vi "Update-PV.vi"(8 "error in (no error)":errorcluster, 10 "PV":refnum<class "PV.lvclass">, 11 "CS++DIM-Client in":refnum<class "CS++DIM-Client.lvclass">) -> (0 "error out":errorcluster, 3 "CS++DIM-Client out":refnum<class "CS++DIM-Client.lvclass">)   [LabVIEW 2014, in "CS++DIM-Client.lvlib" / "CS++DIM-Client.lvclass"]
doc: "Send PV to Actor Core.vi."
uses:
  CS++DIM-Client.lvclass
  CSPP_Core/Classes/CS++ProcessVariables/ProcessVariable/PV.lvclass
  CS++DIM-Client.lvclass/CS++DIM-Client.ctl
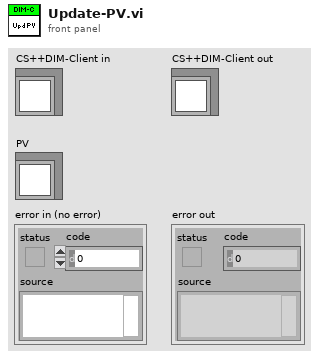
[diagram p1: front panel]
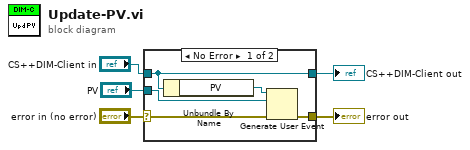
[diagram p0: block diagram]
diagram:
  n1 = case shown="No Error" "error in (no error)" {
    selector: "error in (no error)" -> [w7 w12]
    tunnel: [w6 w12] -> w4
    tunnel: [w10 w11] -> w2
    tunnel: "CS++DIM-Client in" -> [w10 w11]
    tunnel: "PV" -> [w8 _]
    frame No Error {
      n2 = Unbundle By Name(w10) -> ("PV"=w9:refnum<user-event>)
      n3 = Generate User Event(user event=w9, event data cluster=w8, error in=w7) -> (error out=w6:errorcluster)  [unwired: 1 in, 1 out]
    }
    frame Error {
    }
  }
  "error out" <- w4
  "CS++DIM-Client out" <- w2
